vi "Conv_POSE2D_Eng_SI.vi"(11 "Err Pose in ENG":T1 {"ROTATION"."SIN" format="%13.4f"; "ROTATION"."COS" format="%13.4f"; "ROTATION"."VALUE" format="%13.4f"; "TRANSLATION"."Y" format="%14.3f"; "TRANSLATION"."X" format="%14.3f"}) -> (3 "Err Pose out SI":T1 {"ROTATION"."SIN" format="%13.4f"; "ROTATION"."COS" format="%13.4f"; "ROTATION"."VALUE" format="%13.4f"; "TRANSLATION"."Y" format="%14.3f"; "TRANSLATION"."X" format="%14.3f"})   [LabVIEW 2019, in "Trajectory_Library.lvlib"]
doc: "Convert POSE from Meters, Radians to Feet, Radains. (Rotation2d is always stored as radians.) (This is really only for external use. All the internal routines use meters and radians.)"
uses:
  Trajectory_Library.lvlib
  TypeDef/POSE2D.ctl
  TypeDef/TRANSLATION2D.ctl
  TypeDef/ROTATION2D.ctl
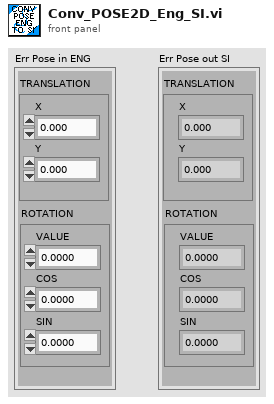
[diagram p1: front panel]
types:
  T1 = typedef "Trajectory_Library.lvlib/POSE2D.ctl" = cluster{"TRANSLATION":T2, "ROTATION":T3}
  T2 = typedef "Trajectory_Library.lvlib/TRANSLATION2D.ctl" = cluster{"X":dbl, "Y":dbl}
  T3 = typedef "Trajectory_Library.lvlib/ROTATION2D.ctl" = cluster{"VALUE":dbl, "COS":dbl, "SIN":dbl}
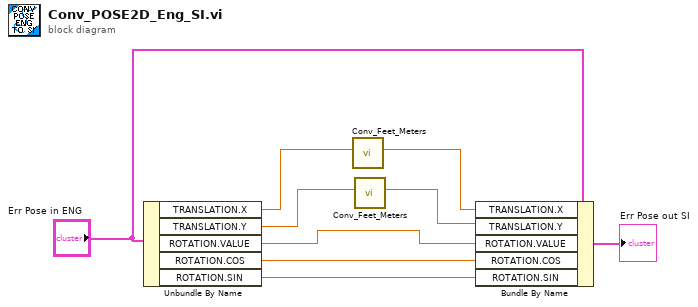
[diagram p0: block diagram]
diagram:
  n1 = Unbundle By Name("Err Pose in ENG") -> ("TRANSLATION.X"=w5:dbl, "TRANSLATION.Y"=w4:dbl, "ROTATION.VALUE"=w1:dbl, "ROTATION.COS"=w7:dbl, "ROTATION.SIN"=w6:dbl)
  n2 = call "Conv_Feet_Meters.vi"("Feet"=w5) -> ("Meters"=w3:dbl)  [unwired: 10 in]
  n3 = call "Conv_Feet_Meters.vi"("Feet"=w4) -> ("Meters"=w2:dbl)  [unwired: 10 in]
  n4 = Bundle By Name(cluster="Err Pose in ENG", "TRANSLATION.X"=w3, "TRANSLATION.Y"=w2, "ROTATION.VALUE"=w1, "ROTATION.COS"=w7, "ROTATION.SIN"=w6) -> (→"Err Pose out SI":T1)
